vi "SetAngleAcceleration.vi"(1 "Time Manager Output":dbl, 2 "Angular Acceleration":dbl) -> (0 "Current Angle":dbl)   [LabVIEW 2015]
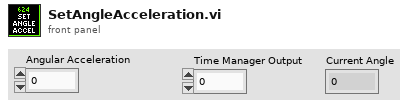
[diagram p1: front panel]
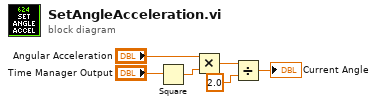
[diagram p0: block diagram]
diagram:
  n1 = Square(x="Time Manager Output") -> (x^2=w4:dbl)
  n2 = Multiply(x="Angular Acceleration", y=w4) -> (x*y=w3:dbl)
  n3 = Divide(x=w3, y=2.0) -> (x/y=→"Current Angle":dbl)
